vi "UpdateImageDisplayGraph.vi"(0 "IntGraph Refnum":refnum<vi>, 1 "X0":dbl, 2 "Y0":dbl, 3 "Width":dbl, 4 "Height":dbl, 5 "# Pixels X":dbl, 6 "# Pixels Y":dbl, 7 "From Center":bool) -> ()   [LabVIEW 2017]
uses:
  <vilib>/express/express arith-compare/Formula/XNode/ExpressFormulaBlockNode.xnode
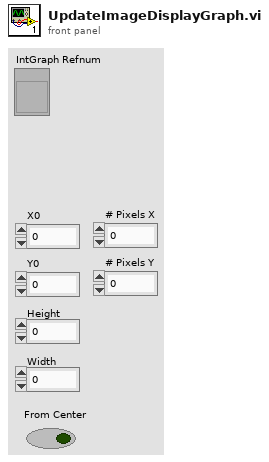
[diagram p1: front panel]
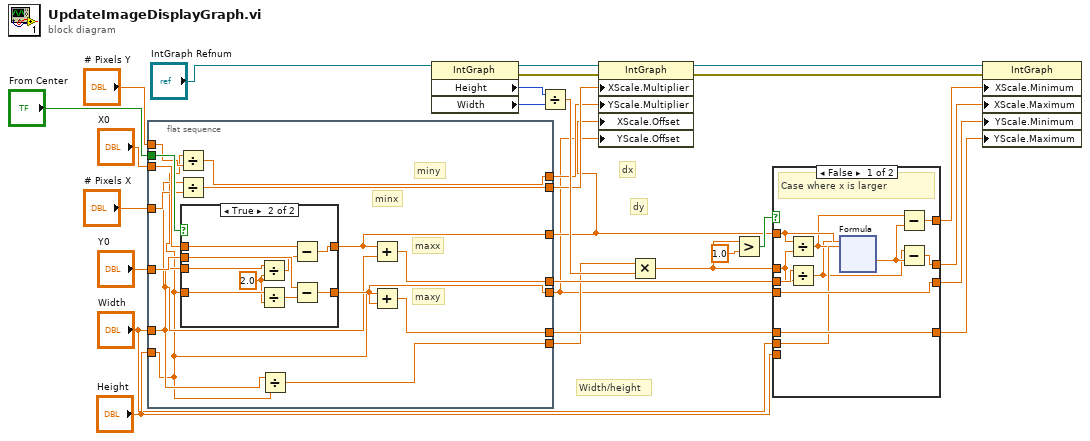
[diagram p0: block diagram]
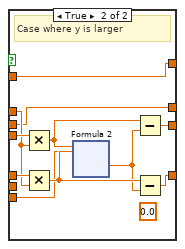
[diagram p3: hidden frame]
diagram:
  # "dy"
  # "dx"
  # "Width/height"
  n1 = flat-sequence {
    tunnel: "# Pixels X" -> [w33]
    tunnel: [w43] -> w14
    tunnel: "# Pixels Y" -> [w32]
    tunnel: [w42] -> w12
    tunnel: "From Center" -> [w41]
    tunnel: "X0" -> [w40]
    tunnel: "Y0" -> [w39]
    tunnel: [w38] -> w3
    tunnel: [w37] -> w8
    tunnel: [w36] -> w2
    tunnel: [w35] -> w7
    tunnel: "Height" -> [w30]
    tunnel: "Width" -> [w31]
    tunnel: [w34] -> w4
    frame #0 {
      # "maxy"
      # "maxx"
      # "miny"
      # "minx"
      n2 = Divide(x=w30, y=w32) -> (x/y=w42:dbl)
      n3 = Divide(x=w31, y=w33) -> (x/y=w43:dbl)
      n4 = case shown="True" w41 {
        tunnel: w40 -> [w45 w49]
        tunnel: w39 -> [w44 w50]
        tunnel: [w45 w47] -> w38
        tunnel: [w44 w46] -> w36
        tunnel: w31 -> [_ w54]
        tunnel: w30 -> [_ w53]
        frame False {
        }
        frame True {
          w52 = 2.0 ("y")
          n5 = Divide(x=w54, y=w52) -> (x/y=w48:dbl)
          n6 = Divide(x=w53, y=w52) -> (x/y=w51:dbl)
          n7 = Subtract(x=w49, y=w48) -> (x-y=w47:dbl)
          n8 = Subtract(x=w50, y=w51) -> (x-y=w46:dbl)
        }
      }
      n9 = Divide(x=w31, y=w30) -> (x/y=w34:dbl)
      n10 = Add(x=w38, y=w31) -> (x+y=w37:dbl)
      n11 = Add(x=w30, y=w36) -> (x+y=w35:dbl)
    }
  }
  n12 = property class="IntGraph"(reference="IntGraph Refnum") -> (reference out=w16:refnum<vi>, error out=w17:errorcluster, "Height"=w29:u32, "Width"=w28:u32)  [unwired: 1 in]
  n13 = Divide(x=w29, y=w28) -> (x/y=w19:dbl)
  n14 = property class="IntGraph"(reference=w16, error in=w17, "XScale.Multiplier"=w14, "YScale.Multiplier"=w12, "XScale.Offset"=w3, "YScale.Offset"=w2) -> (reference out=w25:refnum<vi>, error out=w24:errorcluster)
  n15 = Multiply(x=w4, y=w19) -> (x*y=w18:dbl)
  n16 = Greater?(x=w18, y=1.0) -> (0:w26:bool)
  n17 = case shown="False" w26 {
    tunnel: [w61 w87] -> w23
    tunnel: [w63 w81] -> w21
    tunnel: [w60 w86] -> w22
    tunnel: [w62 w82] -> w20
    tunnel: w3 -> [w58 w87]
    tunnel: w8 -> [w65 w86]
    tunnel: w2 -> [w63 w90]
    tunnel: w7 -> [w62 w89]
    tunnel: w18 -> [w64 w88]
    tunnel: "Height" -> [_ w83]
    tunnel: "Width" -> [w59 _]
    frame False {
      # "Case where x is larger"
      n18 = Divide(x=w58, y=w64) -> (x/y=w56:dbl)
      n19 = Divide(x=w65, y=w64) -> (x/y=w55:dbl)
      n20 = xnode "Formula"("min"=w58, "l"=w59, "minR"=w56, "maxR"=w55) -> ("Result"=w57:dbl)  [unwired: 1 in, 1 out]
      n21 = Subtract(x=w56, y=w57) -> (x-y=w61:dbl)
      n22 = Subtract(x=w55, y=w57) -> (x-y=w60:dbl)
    }
    frame True {
      (unwired) 0.0 ("Y Scale.Offset and Multiplier:Offset")
      # "Case where y is larger"
      n23 = Multiply(x=w90, y=w88) -> (x*y=w85:dbl)
      n24 = Multiply(x=w89, y=w88) -> (x*y=w84:dbl)
      n25 = xnode "Formula 2"("min"=w85, "max"=w84, "l"=w83) -> ("Result"=w80:dbl)  [unwired: 1 in, 1 out]
      n26 = Subtract(x=w85, y=w80) -> (x-y=w81:dbl)
      n27 = Subtract(x=w84, y=w80) -> (x-y=w82:dbl)
    }
  }
  n28 = property class="IntGraph"(reference=w25, error in=w24, "XScale.Minimum"=w23, "XScale.Maximum"=w22, "YScale.Minimum"=w21, "YScale.Maximum"=w20) -> ()  [unwired: 2 out]
